vi "ma_Updatet0 timestamp.vi"(2 "samples":i32, 3 "sampling rate (S/s)":dbl format="%0.2f", 4 "tf previous":timestamp format="%<%.4X>T", 5 "Reset Generation":bool) -> (0 "tf new":timestamp format="%<%.4X>T", 1 "t0":timestamp format="%<%.4X>T")   [LabVIEW 2009]
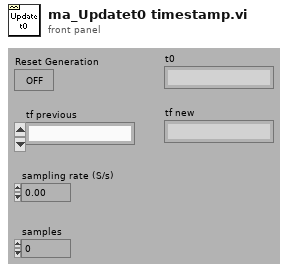
[diagram p1: front panel]
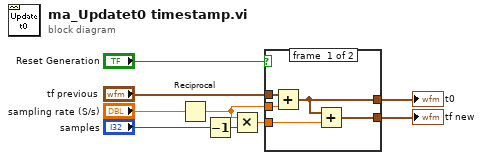
[diagram p0: block diagram]
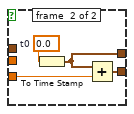
[diagram p2: hidden frame]
diagram:
  n1 = Reciprocal(x="sampling rate (S/s)") -> (1/x=w7:dbl)
  n2 = Decrement(x="samples") -> (x-1=w3:i32)
  n3 = Multiply(x=w7, y=w3) -> (x*y=w4:dbl)
  n4 = case shown="False" "Reset Generation" {
    tunnel: "tf previous" -> [w14 _]
    tunnel: [w13 w17] -> w8
    tunnel: w7 -> [w11 _]
    tunnel: w4 -> [w10 w16]
    tunnel: [w12 w15] -> w2
    frame #0 {
      n5 = Add(x=w14, y=w11) -> (x+y=w13:timestamp)
      n6 = Add(x=w13, y=w10) -> (x+y=w12:timestamp)
    }
    frame #1 {
      w18 = 0.0  # t0
      n7 = To Time Stamp(1:w18) -> (0:w17:timestamp)
      n8 = Add(x=w17, y=w16) -> (x+y=w15:timestamp)
    }
  }
  "t0" <- w8
  "tf new" <- w2
